vi "disdrometer_plotpdfs.vi"(8 "Data B":dbl[](array[numeric]), 9 "Bins B":dbl[](array[numeric]), 10 "Data A":dbl[](array[numeric]), 11 "Bins A":dbl[](array[numeric])) -> (0 "Nb":dbl, 1 "PDF B":cluster{dbl[], dbl[]}, 2 "Na":dbl, 3 "PDF A":cluster{dbl[], dbl[]})   [LabVIEW 2018]
doc: "Used to plot disdrometer PDF results. Takes the bin values and number of observations and formats them into a plot of the percentage of occurences in each bin for the data set.\n\nDoes NOT calculate the PDFs."
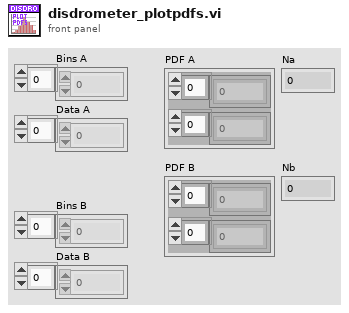
[diagram p1: front panel]
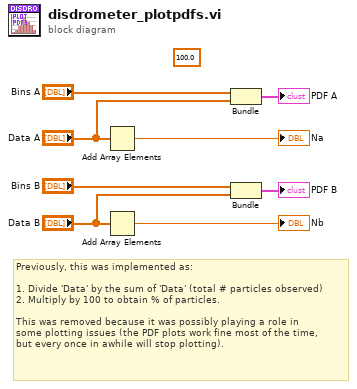
[diagram p0: block diagram]
diagram:
  (unwired) 100.0
  # "Previously, this was implemented as:\n\n1. Divide 'Data' by the sum of 'Data' (total # particles observed)\n2. Multiply by 100 to obtain % of particles.\n\nThis was removed because it was possibly playing a role in\nsome plotting issues (the PDF plots work fine most of the time,\nbut every once in awhile will stop plotting)."
  n1 = Add Array Elements(numeric array="Data A") -> (sum=→"Na":dbl)
  n2 = Add Array Elements(numeric array="Data B") -> (sum=→"Nb":dbl)
  n3 = Bundle("Bins A"="Bins A", "Data A"="Data A") -> (→"PDF A":cluster{"Bins A":dbl[], "Data A":dbl[]})  [unwired: 1 in]
  n4 = Bundle("Bins B"="Bins B", "Data B"="Data B") -> (→"PDF B":cluster{"Bins B":dbl[], "Data B":dbl[]})  [unwired: 1 in]
